vi "ep_Speed Estimation for SVAF.vi"(0 "SVAF spectrum":cluster{"f0":dbl, "df":dbl, "spectrum":dbl[]}, 5 "fundamental frequency [Hz]":dbl format="%#_13g", 7 "nominal frequency":enum16{"50 Hz", "60 Hz"}(ring), 9 "nameplate speed":T1, 11 "error in (no error)":errorcluster, 12 "last valid window":i32) -> (4 "speed data":cluster{"speed [RPM]":dbl, "slip":dbl}={"speed [RPM]"=nan, "slip"=nan}, 14 "current valid window":i32, 15 "error out":errorcluster)   [LabVIEW 2014, in "NI_EP_Motor Monitoring.lvlib"]
uses:
  <vilib>/addons/Electrical Power/Motor Monitoring/NI_EP_Motor Monitoring.lvlib
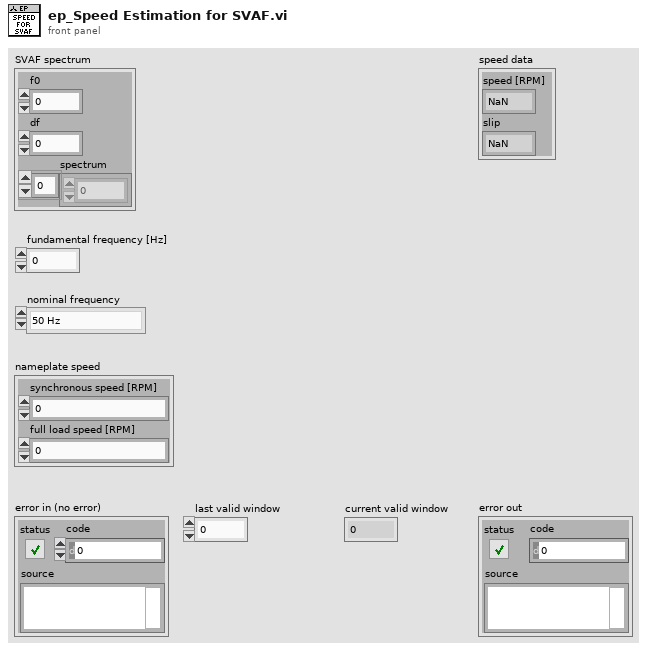
[diagram p1: front panel]
types:
  T1 = cluster{"synchronous speed [RPM]":dbl, "full load speed [RPM]":dbl}
  T2 = cluster{"frequency":dbl[], "magnitude [dB]":dbl[]}
  T3 = cluster{"frequency in window":dbl[], "magnitude in window":dbl[], "enough points for peak search?":bool, "max magnitude in window":dbl}[]
  T4 = cluster{"maximum speed":dbl, "minimum speed":dbl}
  T5 = cluster{"original peak frequency":dbl[], "fitted peak frequency":dbl[], "fitted peak magnitude":dbl[]}[]
  T6 = typedef "NI_EP_Motor Monitoring.lvlib/ep_Harmonic for Speed Calculation.ctl" = enum16{"invalid", "fr", "2fs-2fr", "2fs-fr", "2fr"}
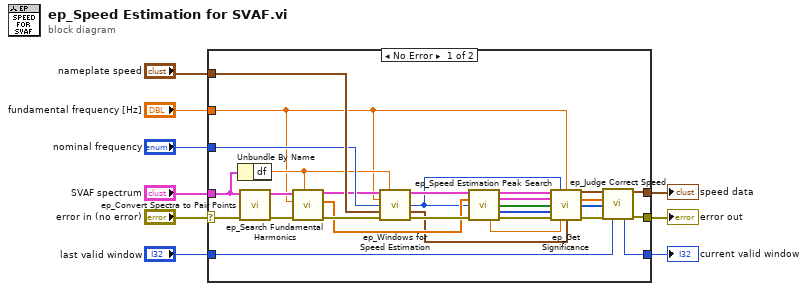
[diagram p0: block diagram]
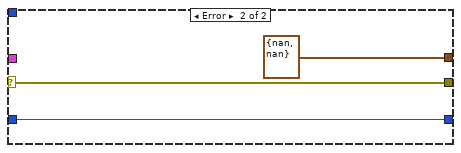
[diagram p2: hidden frame]
diagram:
  n1 = case shown="No Error" "error in (no error)" {
    selector: "error in (no error)" -> [w32 w41]
    tunnel: [w24 w41] -> w8
    tunnel: "fundamental frequency [Hz]" -> [w12 _]
    tunnel: "nameplate speed" -> [w38 _]
    tunnel: "SVAF spectrum" -> [w28 _]
    tunnel: [w23 cluster{"speed [RPM]":dbl, "slip":dbl} {"speed [RPM]"=nan, "slip"=nan} ("speed data")] -> w5
    tunnel: "nominal frequency" -> [w30 _]
    tunnel: "last valid window" -> [w18 w39]
    tunnel: [w17 w39] -> w1
    frame No Error {
      n2 = Unbundle By Name(w28) -> ("df"=w16:dbl)
      n3 = call <vilib>:"ep_Convert Spectra to Pair Points.vi"("error in (no error)"=w32, "spectra"=w28) -> ("error out"=w31:errorcluster, "spectra points"=w26:T2)  [unwired: 6 in, 2 out]
      n4 = call <vilib>:"ep_Search Fundamental Harmonics.vi"("df"=w16, "error in (no error)"=w31, "fundamental frequency [Hz]"=w12, "all spectra points"=w26) -> ("error out"=w37:errorcluster, "fundamental harmonics frequencies"=w15:dbl[], "dup all spectra points"=w29:cluster{"frequency":dbl[], "magnitude":dbl[]})  [unwired: 5 in]
      n5 = call <vilib>:"ep_Windows for Speed Estimation.vi"("all spectra points"=w29, "df"=w16, "fundamental frequency [Hz]"=w12, "nominal frequency"=w30, "nameplate speed"=w38, "error in (no error)"=w37) -> ("points in window"=w27:T3, "pole pairs"=w13:i32, "range of speed"=w11:T4, "error out"=w36:errorcluster)  [unwired: 6 in]
      n6 = call <vilib>:"ep_Speed Estimation Peak Search.vi"("spectra points in window"=w27, "frequencies excluded"=w15, "pole pairs"=w13, "error in (no error)"=w36) -> ("dup spectra points in window"=w35:T3, "peaks information"=w34:T5, "enough points for peak search?"=w22:bool[], "number of peaks"=w21:i32[], "minimum max-magnitude"=w10:dbl, "error out"=w33:errorcluster)  [unwired: 6 in]
      n7 = call <vilib>:"ep_Get Significance.vi"("spectra points in window"=w35, "pole pairs"=w13, "fundamental frequency [Hz]"=w12, "peaks information"=w34, "enough points for peak search?"=w22, "number of peaks"=w21, "error in (no error)"=w33, "minimum max-magnitude"=w10, "range of speed"=w11) -> ("top3 speed data"=w14:cluster{"speed [RPM]":dbl, "slip":dbl}[], "top3 significance"=w20:dbl[], "top3 harmonic for speed calculation"=w19:T6[], "error out"=w25:errorcluster)  [unwired: 3 in]
      n8 = call <vilib>:"ep_Judge Correct Speed.vi"("top3 speed data"=w14, "top3 significance"=w20, "top3 harmonic for speed calculation"=w19, "error in (no error)"=w25, "last valid window"=w18) -> ("speed data"=w23:cluster{"speed [RPM]":dbl, "slip":dbl}, "current valid window"=w17:i32, "error out"=w24:errorcluster)  [unwired: 8 in]
    }
    frame Error {
    }
  }
  "error out" <- w8
  "speed data" <- w5
  "current valid window" <- w1
